vi "Test_Queue.vi"() -> (2 "Tests":cluster{"Test":string, "Passed":bool}[](array[cluster]), 3 "All Passed":bool)   [LabVIEW 2021]
uses:
  ebf6e7bd-4dea-41aa-a4d7-fcabb33fb88a.vi
  1f9cc325-9937-42ad-93f6-0991476be0d9.vi
  af2474c4-2a42-4373-a4e7-d7174c4c717d.vi
  fb02bb9d-60fe-4efe-999d-8fafea34c26a.vi
  86eb2c31-2ef4-4f52-8c7e-c4cd79eee94b.vi
  15bb192a-e047-4910-b6c7-e2d91b4fb920.vi
  e3e0b692-3f05-4cc3-bcdb-d52b2cb1c00c.vi
  07afb981-15fc-4acc-97a8-0c99b9836663.vi
  0269a72d-fd89-4c26-9187-e43185b182b9.vi
  803f4470-47be-4643-a591-48d54bf1cc4c.vi
  ec5fa7b9-9761-43ce-ad51-dc8d7309023d.vi
  7d11f8f4-9aa5-40e4-88f9-cf15113ac809.vi
  a4e05b25-b2fd-4a62-9474-6c8b1c6ba464.vi
  3a933310-1996-4eb1-bb35-2cef4bbc9920.vi
  3fbf7aaa-d5ae-4bec-ab0e-4ac27ad070b2.vi
  f4553291-fa86-418b-b39e-46cdf70e043e.vi
  b3874ef4-d7c0-4545-bae3-25086f4fe7ad.vi
  1ab1bd47-603c-456c-b9d0-96944e88f92c.vi
  ebbe48c1-b72b-4de3-aeb3-ba80bb7d0d19.vi
  8bdc6467-f6e5-4f75-9ac6-95094b1edd2b.vi
  35eb1fc5-534c-4ae0-b18f-a29eee8d1686.vi
  14dfade2-853f-44e8-b475-1791b1f25eec.vi
  4af17a5a-468f-4981-8f40-38f2c589f87d.vi
  fafea8c6-e71b-47bf-8fdc-74539dc463ec.vi
  be416df7-4f26-4020-a28b-5e551047e503.vi
  8d7d29ec-df87-4bcc-9fa1-3aa083bb282c.vi
  6a558a1d-279f-4cd8-a1d4-0ce029900aa4.vi
  7b643780-0266-49a5-bff5-7ddf02e75eca.vi
  b89bb2c3-d50e-4ca1-96dc-4f6891fa975b.vi
  f7c266ed-5b2f-4925-8a7e-d3378c7bde95.vi
  22155a5e-7ba0-482a-9fa4-40093b810291.vi
  <vilib>/Utility/error.llb/Error Cluster From Error Code.vi
  src/SubVIs/Map.vi
  src/Queue.lvlib
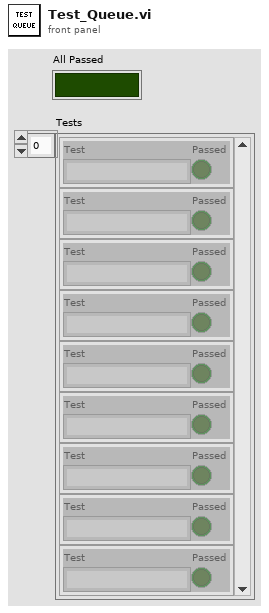
[diagram p1: front panel]
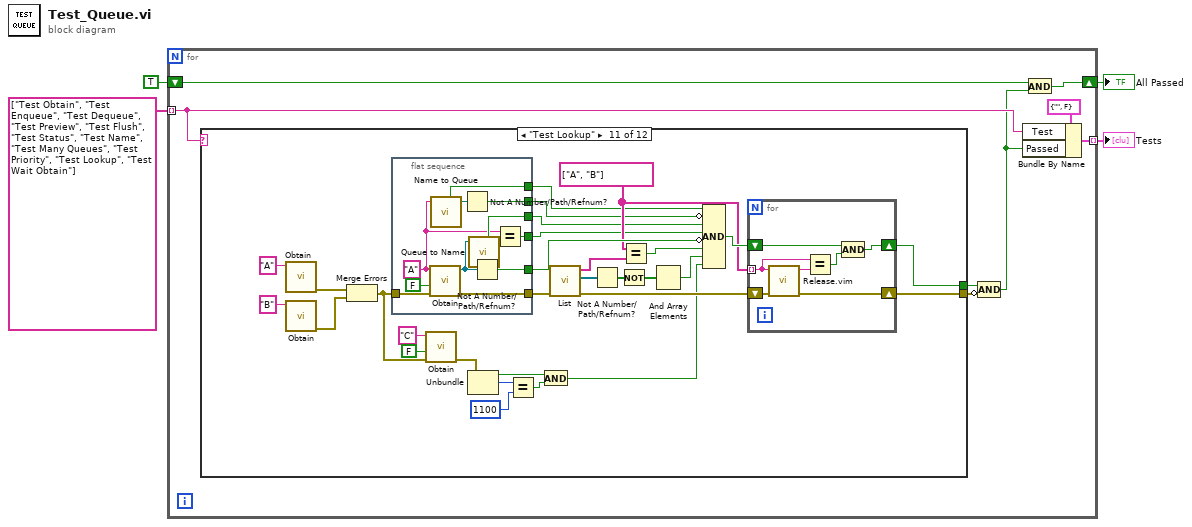
[diagram p0: block diagram]
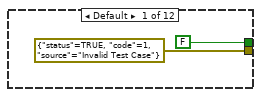
[diagram p2: hidden frame]
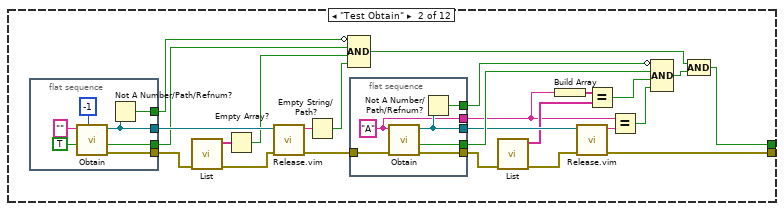
[diagram p3: hidden frame]
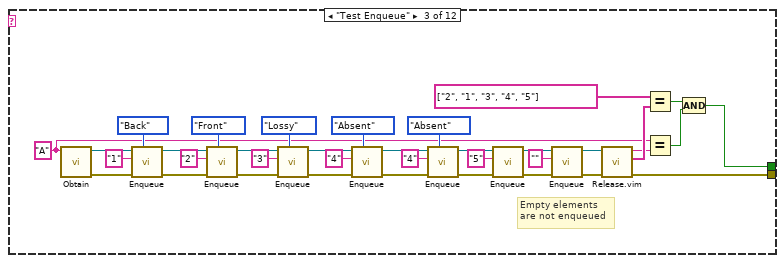
[diagram p4: hidden frame]
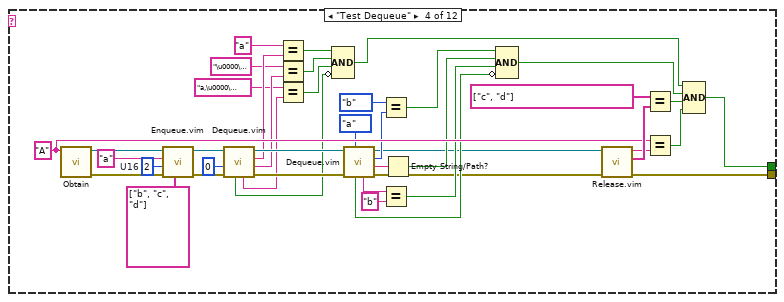
[diagram p5: hidden frame]
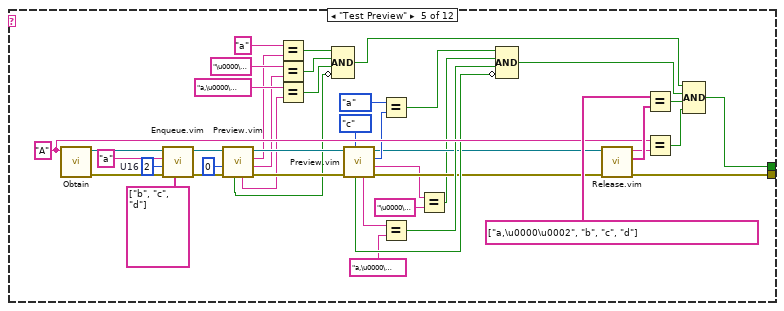
[diagram p6: hidden frame]
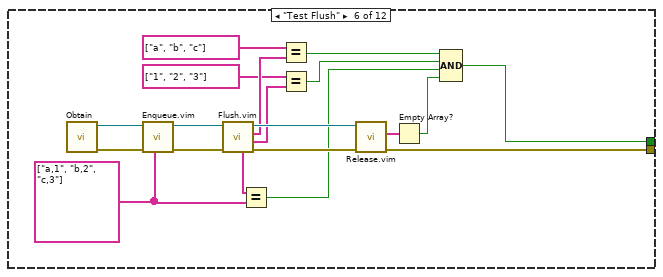
[diagram p7: hidden frame]
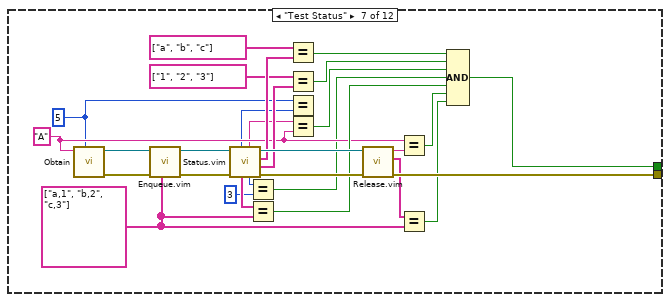
[diagram p8: hidden frame]
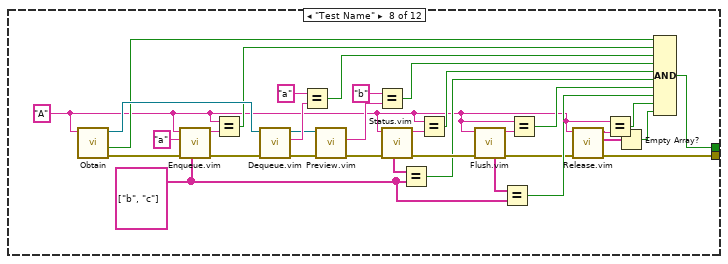
[diagram p9: hidden frame]
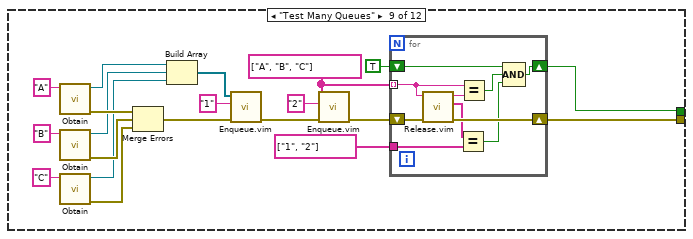
[diagram p10: hidden frame]
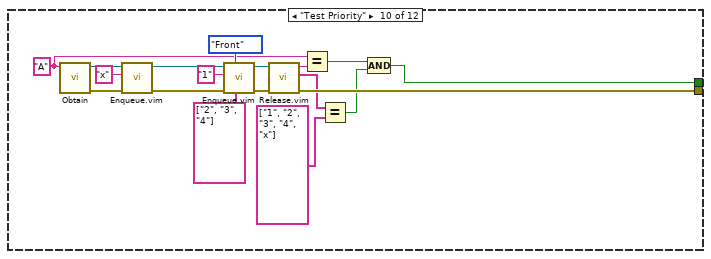
[diagram p11: hidden frame]
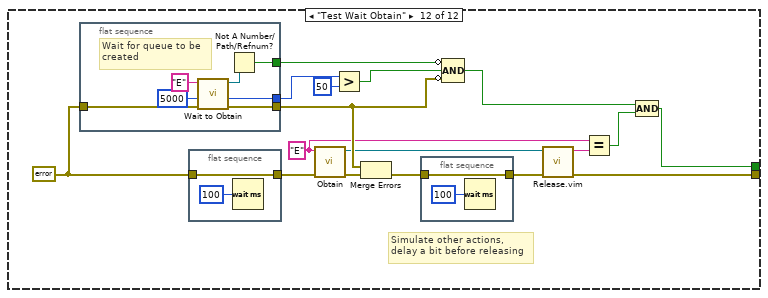
[diagram p12: hidden frame]
diagram:
  n1 = for {
    tunnel: string[] ["Test Obtain", "Test Enqueue", "Test Dequeue", "Test Preview", "Test Flush", "Test Status", "Test Name", "Test Many Queues", "Test Priority", "Test Lookup", "Test Wait Obtain"] -> [w8] mode=indexing
    shift-right: [w10] -> w2
    shift-left: TRUE -> [w11]
    tunnel: [w9] -> w1 mode=indexing
    n2 = case shown="\"Test Lookup\"" w8 {
      tunnel: [FALSE w30 w64 w126 w169 w180 w213 w222 w256 w291 w331 w358] -> w7
      tunnel: [errorcluster {"status"=TRUE, "code"=1, "source"="Invalid Test Case"} ("error in (no error)") w29 w67 w129 w172 w192 w221 w223 w260 w298 w333 w363] -> w5
      frame Default {
      }
      frame "Test Obtain" {
        n3 = flat-sequence {
          tunnel: [w52] -> w24
          tunnel: [w50] -> w39
          tunnel: [w49] -> w38
          tunnel: [w48] -> w37
          frame #0 {
            n4 = call "Obtain.vi"("Max Size (-1=Unlimited)"=-1, "Create if not Found? (T)"=TRUE, "Queue Name (\"\"=Unnamed)"="" ("Queue Name (\"\"=Unnamed)")) -> ("error out"=w52:errorcluster, "Created New?"=w48:bool, "Queue out"=w50:refnum<queue>)  [unwired: 6 in]
            n5 = Not A Number/Path/Refnum?(number/path/refnum=w50) -> (NaN/Path/Refnum?=w49:bool)
          }
        }
        n6 = call "List.vi"("error in (no error)"=w24) -> ("error out"=w23:errorcluster, "Queue Names"=w22:string[])  [unwired: 8 in, 1 out]
        n7 = Empty Array?(array=w22) -> (empty?=w21:bool)
        n8 = call "Release.vim"("error in (no error)"=w23, "Queue in"=w39) -> ("error out"=w33:errorcluster, "Queue Name"=w26:string)  [unwired: 7 in, 1 out]
        n9 = Empty String/Path?(string/path=w26) -> (empty?=w25:bool)
        n10 = Compound Arithmetic op=AND(invert w38, w37, w21, w25) -> (w31:bool)
        n11 = flat-sequence {
          tunnel: [w45] -> w36
          tunnel: [w44] -> w35
          tunnel: [w43] -> w34
          tunnel: [w42] -> w20
          tunnel: w33 -> [w41]
          tunnel: [w40] -> w16
          frame #0 {
            w40 = "A" ("Queue Name (\"\"=Unnamed)")
            n12 = call "Obtain.vi"("error in (no error)"=w41, "Queue Name (\"\"=Unnamed)"=w40) -> ("error out"=w42:errorcluster, "Created New?"=w45:bool, "Queue out"=w43:refnum<queue>)  [unwired: 7 in]
            n13 = Not A Number/Path/Refnum?(number/path/refnum=w43) -> (NaN/Path/Refnum?=w44:bool)
          }
        }
        n14 = call "List.vi"("error in (no error)"=w20) -> ("error out"=w19:errorcluster, "Queue Names"=w18:string[])  [unwired: 8 in, 1 out]
        n15 = Build Array(w16) -> (w17:string[])
        n16 = call "Release.vim"("error in (no error)"=w19, "Queue in"=w34) -> ("error out"=w29:errorcluster, "Queue Name"=w28:string)  [unwired: 7 in, 1 out]
        n17 = Equal?(x=w17, y=w18) -> (x = y?=w15:bool)
        n18 = Equal?(x=w16, y=w28) -> (x = y?=w27:bool)
        n19 = Compound Arithmetic op=AND(invert w35, w36, w15, w27) -> (w32:bool)
        n20 = Compound Arithmetic op=AND(w31, w32) -> (w30:bool)
      }
      frame "Test Enqueue" {
        w61 = "A" ("Queue Name (\"\"=Unnamed)")
        # "Empty elements\nare not enqueued"
        n21 = call "Obtain.vi"("Queue Name (\"\"=Unnamed)"=w61) -> ("error out"=w87:errorcluster, "Queue out"=w88:refnum<queue>)  [unwired: 8 in, 1 out]
        n22 = call "Enqueue.vi"("Method (Back)"=enum8{"Back", "Front", "Lossy", "Absent"}."Back", "error in (no error)"=w87, "Element"="1", "Queue in"=w88) -> ("error out"=w81:errorcluster, "Queue out"=w82:refnum<queue>)  [unwired: 6 in]
        n23 = call "Enqueue.vi"("Method (Back)"=enum8{"Back", "Front", "Lossy", "Absent"}."Front", "error in (no error)"=w81, "Element"="2", "Queue in"=w82) -> ("error out"=w77:errorcluster, "Queue out"=w78:refnum<queue>)  [unwired: 6 in]
        n24 = call "Enqueue.vi"("Method (Back)"=enum8{"Back", "Front", "Lossy", "Absent"}."Lossy", "error in (no error)"=w77, "Element"="3", "Queue in"=w78) -> ("error out"=w73:errorcluster, "Queue out"=w74:refnum<queue>)  [unwired: 6 in]
        n25 = call "Enqueue.vi"("Method (Back)"=enum8{"Back", "Front", "Lossy", "Absent"}."Absent", "error in (no error)"=w73, "Element"="4", "Queue in"=w74) -> ("error out"=w69:errorcluster, "Queue out"=w70:refnum<queue>)  [unwired: 6 in]
        n26 = call "Enqueue.vi"("Method (Back)"=enum8{"Back", "Front", "Lossy", "Absent"}."Absent", "error in (no error)"=w69, "Element"="4", "Queue in"=w70) -> ("error out"=w59:errorcluster, "Queue out"=w60:refnum<queue>)  [unwired: 6 in]
        n27 = call "Enqueue.vi"("error in (no error)"=w59, "Element"="5", "Queue in"=w60) -> ("error out"=w56:errorcluster, "Queue out"=w57:refnum<queue>)  [unwired: 7 in]
        n28 = call "Enqueue.vi"("error in (no error)"=w56, "Element"="", "Queue in"=w57) -> ("error out"=w55:errorcluster, "Queue out"=w54:refnum<queue>)  [unwired: 7 in]
        n29 = call "Release.vim"("error in (no error)"=w55, "Queue in"=w54) -> ("error out"=w67:errorcluster, "Remaining Elements"=w66:string[], "Queue Name"=w63:string)  [unwired: 7 in]
        n30 = Equal?(x=string[] ["2", "1", "3", "4", "5"] ("y"), y=w66) -> (x = y?=w65:bool)
        n31 = Equal?(x=w61, y=w63) -> (x = y?=w62:bool)
        n32 = Compound Arithmetic op=AND(w65, w62) -> (w64:bool)
      }
      frame "Test Dequeue" {
        w119 = u16 2  # U16
        w123 = "A" ("Queue Name (\"\"=Unnamed)")
        n33 = call "Obtain.vi"("Queue Name (\"\"=Unnamed)"=w123) -> ("error out"=w121:errorcluster, "Queue out"=w122:refnum<queue>)  [unwired: 8 in, 1 out]
        n34 = call "Enqueue.vim"("Messages"=string[] ["b", "c", "d"], "error in (no error)"=w121, "Data"=w119, "Message"="a", "Queue in"=w122) -> ("error out"=w117:errorcluster, "Queue out"=w116:refnum<queue>)  [unwired: 5 in]
        n35 = call "Dequeue.vim"("error in (no error)"=w117, "Timeout in ms (-1)"=0, "Queue in"=w116) -> ("error out"=w114:errorcluster, "Data"=w110:string, "Message"=w112:string, "Queue out"=w113:refnum<queue>, "Element"=w105:string, "Timed Out?"=w103:bool)  [unwired: 3 in]
        n36 = Equal?(x="a", y=w112) -> (x = y?=w108:bool)
        n37 = Equal?(x="\u0000\u0002", y=w110) -> (x = y?=w107:bool)
        n38 = Equal?(x="a,\u0000\u0002", y=w105) -> (x = y?=w104:bool)
        n39 = Compound Arithmetic op=AND(w108, w107, w104, invert w103) -> (w89:bool)
        n40 = call "Dequeue.vim"("Message Type"=enum16{"a", "b", "c", "d"}."a", "error in (no error)"=w114, "Queue in"=w113) -> ("error out"=w92:errorcluster, "Data"=w98:string, "Message"=w101:enum16{"a", "b", "c", "d"}, "Queue out"=w91:refnum<queue>, "Element"=w96:string, "Timed Out?"=w93:bool)  [unwired: 3 in]
        n41 = Equal?(x=enum16{"a", "b", "c", "d"}."b", y=w101) -> (x = y?=w99:bool)
        n42 = Equal?(x=w96, y="b") -> (x = y?=w94:bool)
        n43 = Empty String/Path?(string/path=w98) -> (empty?=w97:bool)
        n44 = Compound Arithmetic op=AND(w99, w97, w94, invert w93) -> (w90:bool)
        n45 = call "Release.vim"("error in (no error)"=w92, "Queue in"=w91) -> ("error out"=w129:errorcluster, "Remaining Elements"=w128:string[], "Queue Name"=w125:string)  [unwired: 7 in]
        n46 = Equal?(x=string[] ["c", "d"] ("y"), y=w128) -> (x = y?=w127:bool)
        n47 = Equal?(x=w123, y=w125) -> (x = y?=w124:bool)
        n48 = Compound Arithmetic op=AND(w89, w90, w127, w124) -> (w126:bool)
      }
      frame "Test Preview" {
        w162 = u16 2  # U16
        w166 = "A" ("Queue Name (\"\"=Unnamed)")
        n49 = call "Obtain.vi"("Queue Name (\"\"=Unnamed)"=w166) -> ("error out"=w164:errorcluster, "Queue out"=w165:refnum<queue>)  [unwired: 8 in, 1 out]
        n50 = call "Enqueue.vim"("Messages"=string[] ["b", "c", "d"], "error in (no error)"=w164, "Data"=w162, "Message"="a", "Queue in"=w165) -> ("error out"=w143:errorcluster, "Queue out"=w142:refnum<queue>)  [unwired: 5 in]
        n51 = call "Preview.vim"("error in (no error)"=w143, "Timeout in ms (-1)"=0, "Queue in"=w142) -> ("error out"=w140:errorcluster, "Data"=w136:string, "Message"=w135:string, "Queue out"=w141:refnum<queue>, "Element"=w138:string, "Timed Out?"=w137:bool)  [unwired: 3 in]
        n52 = Equal?(x="a", y=w135) -> (x = y?=w158:bool)
        n53 = Equal?(x="\u0000\u0002", y=w136) -> (x = y?=w157:bool)
        n54 = Equal?(x="a,\u0000\u0002", y=w138) -> (x = y?=w155:bool)
        n55 = Compound Arithmetic op=AND(w158, w157, w155, invert w137) -> (w144:bool)
        n56 = call "Preview.vim"("Message Type"=enum16{"a", "b", "c", "d"}."c", "error in (no error)"=w140, "Queue in"=w141) -> ("error out"=w147:errorcluster, "Data"=w132:string, "Message"=w153:enum16{"a", "b", "c", "d"}, "Queue out"=w146:refnum<queue>, "Element"=w150:string, "Timed Out?"=w148:bool)  [unwired: 3 in]
        n57 = Equal?(x=enum16{"a", "b", "c", "d"}."a", y=w153) -> (x = y?=w151:bool)
        n58 = Equal?(x=w150, y="a,\u0000\u0002" ("x")) -> (x = y?=w149:bool)
        n59 = Equal?(x=w132, y="\u0000\u0002" ("x")) -> (x = y?=w131:bool)
        n60 = Compound Arithmetic op=AND(w151, w131, w149, invert w148) -> (w145:bool)
        n61 = call "Release.vim"("error in (no error)"=w147, "Queue in"=w146) -> ("error out"=w172:errorcluster, "Remaining Elements"=w171:string[], "Queue Name"=w168:string)  [unwired: 7 in]
        n62 = Equal?(x=string[] ["a,\u0000\u0002", "b", "c", "d"] ("y"), y=w171) -> (x = y?=w170:bool)
        n63 = Equal?(x=w166, y=w168) -> (x = y?=w167:bool)
        n64 = Compound Arithmetic op=AND(w144, w145, w170, w167) -> (w169:bool)
      }
      frame "Test Flush" {
        w184 = string[] ["a,1", "b,2", "c,3"] ("Messages")
        n65 = call "Obtain.vi"() -> ("error out"=w188:errorcluster, "Queue out"=w189:refnum<queue>)  [unwired: 9 in, 1 out]
        n66 = call "Enqueue.vim"("Messages"=w184, "error in (no error)"=w188, "Queue in"=w189) -> ("error out"=w186:errorcluster, "Queue out"=w187:refnum<queue>)  [unwired: 7 in]
        n67 = call "Flush.vim"("error in (no error)"=w186, "Queue in"=w187) -> ("error out"=w191:errorcluster, "Data"=w176:string[], "Messages"=w179:string[], "Queue out"=w190:refnum<queue>, "Elements"=w185:string[])  [unwired: 5 in]
        n68 = Equal?(x=w185, y=w184) -> (x = y?=w181:bool)
        n69 = Equal?(x=string[] ["a", "b", "c"], y=w179) -> (x = y?=w174:bool)
        n70 = Equal?(x=string[] ["1", "2", "3"], y=w176) -> (x = y?=w175:bool)
        n71 = call "Release.vim"("error in (no error)"=w191, "Queue in"=w190) -> ("error out"=w192:errorcluster, "Remaining Elements"=w183:string[])  [unwired: 7 in, 1 out]
        n72 = Empty Array?(array=w183) -> (empty?=w182:bool)
        n73 = Compound Arithmetic op=AND(w174, w175, w181, w182) -> (w180:bool)
      }
      frame "Test Status" {
        w197 = 5 ("Max Size (-1=Unlimited)")
        w201 = "A" ("Queue Name (\"\"=Unnamed)")
        w204 = string[] ["a,1", "b,2", "c,3"] ("Messages")
        n74 = call "Obtain.vi"("Max Size (-1=Unlimited)"=w197, "Queue Name (\"\"=Unnamed)"=w201) -> ("error out"=w217:errorcluster, "Queue out"=w218:refnum<queue>)  [unwired: 7 in, 1 out]
        n75 = call "Enqueue.vim"("Messages"=w204, "error in (no error)"=w217, "Queue in"=w218) -> ("error out"=w215:errorcluster, "Queue out"=w216:refnum<queue>)  [unwired: 7 in]
        n76 = call "Status.vim"("error in (no error)"=w215, "Queue in"=w216) -> ("error out"=w220:errorcluster, "Data"=w209:string[], "Messages"=w212:string[], "Queue out"=w219:refnum<queue>, "# Elements in Queue"=w196:i32, "Queue Name"=w200:string, "Elements"=w206:string[], "Max Size"=w198:i32)  [unwired: 2 in]
        n77 = Equal?(x=w196, y=3) -> (x = y?=w194:bool)
        n78 = Equal?(x=w206, y=w204) -> (x = y?=w214:bool)
        n79 = Equal?(x=string[] ["a", "b", "c"], y=w212) -> (x = y?=w207:bool)
        n80 = Equal?(x=string[] ["1", "2", "3"], y=w209) -> (x = y?=w208:bool)
        n81 = Equal?(x=w197, y=w198) -> ()  [unwired: 1 out]
        n82 = Equal?(x=w200, y=w201) -> (x = y?=w199:bool)
        n83 = call "Release.vim"("error in (no error)"=w220, "Queue in"=w219) -> ("error out"=w221:errorcluster, "Remaining Elements"=w205:string[], "Queue Name"=w202:string)  [unwired: 7 in]
        n84 = Equal?(x=w201, y=w202) -> (x = y?=w193:bool)
        n85 = Equal?(x=w205, y=w204) -> (x = y?=w203:bool)
        n86 = Compound Arithmetic op=AND(w207, w208, w199, w194, w214, w193, w203) -> (w213:bool)
      }
      frame "Test Name" {
        w232 = string[] ["b", "c"] ("Messages")
        w227 = "A" ("Queue Name (\"\"=Unnamed)")
        n87 = call "Obtain.vi"("Queue Name (\"\"=Unnamed)"=w227) -> ("error out"=w255:errorcluster, "Created New?"=w248:bool, "Queue out"=w252:refnum<queue>)  [unwired: 8 in]
        n88 = call "Enqueue.vim"("Messages"=w232, "error in (no error)"=w255, "Message"="a", "Queue in"=w227) -> ("error out"=w253:errorcluster, "Queue out"=w238:string)  [unwired: 6 in]
        n89 = Equal?(x=w227, y=w238) -> (x = y?=w237:bool)
        n90 = call "Dequeue.vim"("error in (no error)"=w253, "Queue in"=w252) -> ("error out"=w247:errorcluster, "Message"=w251:string, "Queue out"=w246:refnum<queue>)  [unwired: 4 in, 3 out]
        n91 = Equal?(x="a", y=w251) -> (x = y?=w249:bool)
        n92 = call "Preview.vim"("error in (no error)"=w247, "Queue in"=w246) -> ("error out"=w242:errorcluster, "Message"=w244:string)  [unwired: 4 in, 4 out]
        n93 = Equal?(x="b", y=w244) -> (x = y?=w243:bool)
        n94 = call "Status.vim"("error in (no error)"=w242, "Queue in"=w227) -> ("error out"=w241:errorcluster, "Queue out"=w240:string, "Elements"=w236:string[])  [unwired: 2 in, 5 out]
        n95 = Equal?(x=w236, y=w232) -> (x = y?=w234:bool)
        n96 = Equal?(x=w227, y=w240) -> (x = y?=w235:bool)
        n97 = call "Flush.vim"("error in (no error)"=w241, "Queue in"=w227) -> ("error out"=w229:errorcluster, "Queue out"=w239:string, "Elements"=w233:string[])  [unwired: 5 in, 2 out]
        n98 = Equal?(x=w233, y=w232) -> (x = y?=w230:bool)
        n99 = Equal?(x=w227, y=w239) -> (x = y?=w231:bool)
        n100 = call "Release.vim"("error in (no error)"=w229, "Queue in"=w227) -> ("error out"=w223:errorcluster, "Remaining Elements"=w225:string[], "Queue Name"=w228:string)  [unwired: 7 in]
        n101 = Equal?(x=w227, y=w228) -> (x = y?=w226:bool)
        n102 = Empty Array?(array=w225) -> (empty?=w224:bool)
        n103 = Compound Arithmetic op=AND(w248, w237, w249, w243, w235, w234, w231, w230, w226, w224) -> (w222:bool)
      }
      frame "Test Many Queues" {
        w259 = string[] ["A", "B", "C"]
        n104 = call "Obtain.vi"("Queue Name (\"\"=Unnamed)"="A" ("Queue Name (\"\"=Unnamed)")) -> ("error out"=w272:errorcluster, "Queue out"=w265:refnum<queue>)  [unwired: 8 in, 1 out]
        n105 = call "Obtain.vi"("Queue Name (\"\"=Unnamed)"="B" ("Queue Name (\"\"=Unnamed)")) -> ("error out"=w273:errorcluster, "Queue out"=w264:refnum<queue>)  [unwired: 8 in, 1 out]
        n106 = call "Obtain.vi"("Queue Name (\"\"=Unnamed)"="C" ("Queue Name (\"\"=Unnamed)")) -> ("error out"=w270:errorcluster, "Queue out"=w263:refnum<queue>)  [unwired: 8 in, 1 out]
        n107 = Merge Errors(w272, w273, w270) -> (w267:errorcluster)
        n108 = Build Array(w265, w264, w263) -> (w262:refnum<queue>[])
        n109 = call "Enqueue.vim"("error in (no error)"=w267, "Message"="1", "Queue in"=w262) -> ("error out"=w266:errorcluster)  [unwired: 7 in, 1 out]
        n110 = call "Enqueue.vim"("error in (no error)"=w266, "Message"="2", "Queue in"=w259) -> ("error out"=w261:errorcluster)  [unwired: 7 in, 1 out]
        n111 = for {
          shift-right: [w284] -> w260
          shift-left: w261 -> [w285]
          tunnel: w259 -> [w282] mode=indexing
          tunnel: string[] ["1", "2"] ("y") -> [w280]
          shift-right: [w277] -> w256
          shift-left: TRUE -> [w276]
          n112 = call "Release.vim"("error in (no error)"=w285, "Queue in"=w282) -> ("error out"=w284:errorcluster, "Remaining Elements"=w281:string[], "Queue Name"=w283:string)  [unwired: 7 in]
          n113 = Equal?(x=w281, y=w280) -> (x = y?=w278:bool)
          n114 = Equal?(x=w282, y=w283) -> (x = y?=w279:bool)
          n115 = Compound Arithmetic op=AND(w276, w279, w278) -> (w277:bool)
        }
      }
      frame "Test Priority" {
        w295 = "A" ("Queue Name (\"\"=Unnamed)")
        n116 = call "Obtain.vi"("Queue Name (\"\"=Unnamed)"=w295) -> ("error out"=w289:errorcluster, "Queue out"=w290:refnum<queue>)  [unwired: 8 in, 1 out]
        n117 = call "Enqueue.vim"("error in (no error)"=w289, "Message"="x", "Queue in"=w290) -> ("error out"=w288:errorcluster, "Queue out"=w287:refnum<queue>)  [unwired: 7 in]
        n118 = call "Enqueue.vim"("Messages"=string[] ["2", "3", "4"], "Method (Back)"=enum8{"Back", "Front", "Lossy", "Absent"}."Front", "error in (no error)"=w288, "Message"="1", "Queue in"=w287) -> ("error out"=w300:errorcluster, "Queue out"=w299:refnum<queue>)  [unwired: 5 in]
        n119 = call "Release.vim"("error in (no error)"=w300, "Queue in"=w299) -> ("error out"=w298:errorcluster, "Remaining Elements"=w297:string[], "Queue Name"=w296:string)  [unwired: 7 in]
        n120 = Equal?(x=w295, y=w296) -> (x = y?=w293:bool)
        n121 = Equal?(x=w297, y=string[] ["1", "2", "3", "4", "x"]) -> (x = y?=w292:bool)
        n122 = Compound Arithmetic op=AND(w293, w292) -> (w291:bool)
      }
      frame "Test Lookup" {
        w308 = string[] ["A", "B"] ("y")
        n123 = call "Obtain.vi"("Queue Name (\"\"=Unnamed)"="A" ("Queue Name (\"\"=Unnamed)")) -> ("error out"=w330:errorcluster)  [unwired: 8 in, 2 out]
        n124 = call "Obtain.vi"("Queue Name (\"\"=Unnamed)"="B" ("Queue Name (\"\"=Unnamed)")) -> ("error out"=w328:errorcluster)  [unwired: 8 in, 2 out]
        n125 = Merge Errors(w330, w328) -> (w325:errorcluster)
        n126 = flat-sequence {
          tunnel: w325 -> [w351]
          tunnel: [w350] -> w319
          tunnel: [w349] -> w318
          tunnel: [w347] -> w307
          tunnel: [w346] -> w306
          tunnel: [w344] -> w305
          tunnel: [w341] -> w304
          frame #0 {
            w342 = "A" ("Queue Name (\"\"=Unnamed)")
            n127 = call "Obtain.vi"("error in (no error)"=w351, "Create if not Found? (T)"=FALSE, "Queue Name (\"\"=Unnamed)"=w342) -> ("error out"=w349:errorcluster, "Queue out"=w345:refnum<queue>)  [unwired: 6 in, 1 out]
            n128 = call "Name to Queue.vi"("Queue Name in"=w342) -> ("Found?"=w346:bool, "Queue out"=w348:refnum<queue>)  [unwired: 7 in]
            n129 = Not A Number/Path/Refnum?(number/path/refnum=w348) -> (NaN/Path/Refnum?=w347:bool)
            n130 = call "Queue to Name.vi"("Queue in"=w345) -> ("Found?"=w344:bool, "Queue Name out"=w343:string)  [unwired: 7 in]
            n131 = Not A Number/Path/Refnum?(number/path/refnum=w345) -> (NaN/Path/Refnum?=w350:bool)
            n132 = Equal?(x=w342, y=w343) -> (x = y?=w341:bool)
          }
        }
        n133 = call "Obtain.vi"("error in (no error)"=w325, "Create if not Found? (T)"=FALSE, "Queue Name (\"\"=Unnamed)"="C" ("Queue Name (\"\"=Unnamed)")) -> ("error out"=w324:errorcluster)  [unwired: 6 in, 2 out]
        n134 = Unbundle(w324) -> ("status"=w322:bool, "code"=w323:i32)  [unwired: 1 out]
        n135 = Equal?(x=w323, y=1100) -> (x = y?=w321:bool)
        n136 = And(x=w322, y=w321) -> (x .and. y?=w315:bool)
        n137 = call "List.vi"("error in (no error)"=w318) -> ("error out"=w316:errorcluster, "Queues"=w313:refnum<queue>[], "Queue Names"=w314:string[])  [unwired: 8 in]
        n138 = Not A Number/Path/Refnum?(number/path/refnum=w313) -> (NaN/Path/Refnum?=w312:bool[])
        n139 = Not(x=w312) -> (.not. x?=w311:bool[])
        n140 = Equal?(x=w308, y=w314) -> (x = y?=w317:bool)
        n141 = And Array Elements(Boolean array=w311) -> (logical AND=w310:bool)
        n142 = Compound Arithmetic op=AND(w306, invert w307, w305, w304, invert w319, w317, w310, w315) -> (w309:bool)
        n143 = for {
          shift-right: [w340] -> w333
          shift-left: w316 -> [w336]
          shift-right: [w337] -> w331
          shift-left: w309 -> [w335]
          tunnel: w308 -> [w334] mode=indexing
          n144 = call "Release.vim"("error in (no error)"=w336, "Queue in"=w334) -> ("error out"=w340:errorcluster, "Queue Name"=w339:string)  [unwired: 7 in, 1 out]
          n145 = Equal?(x=w334, y=w339) -> (x = y?=w338:bool)
          n146 = Compound Arithmetic op=AND(w335, w338) -> (w337:bool)
        }
      }
      frame "Test Wait Obtain" {
        w369 = errorcluster {"status"=FALSE, "code"=0, "source"=""} ("error in (no error)")
        w361 = "E" ("Queue Name (\"\"=Unnamed)")
        # "Simulate other actions,\ndelay a bit before releasing"
        n147 = flat-sequence {
          tunnel: w369 -> [w377]
          tunnel: [w374] -> w367
          tunnel: [w373] -> w365
          tunnel: [w372] -> w357
          frame #0 {
            # "Wait for queue to be\ncreated"
            n148 = call "Wait to Obtain.vi"("error in (no error)"=w377, "Timeout in ms (5000)"=u32 5000, "Queue Name"="E") -> ("error out"=w373:errorcluster, "ms Elapsed"=w372:u32, "Queue out"=w375:refnum<queue>)  [unwired: 6 in]
            n149 = Not A Number/Path/Refnum?(number/path/refnum=w375) -> (NaN/Path/Refnum?=w374:bool)
          }
        }
        n150 = flat-sequence {
          tunnel: w369 -> [w379]
          tunnel: [w379] -> w368
          frame #0 {
            n151 = Wait (ms)(milliseconds to wait=u32 100) -> ()  [unwired: 1 out]
          }
        }
        n152 = call "Obtain.vi"("error in (no error)"=w368, "Queue Name (\"\"=Unnamed)"=w361) -> ("error out"=w366:errorcluster, "Queue out"=w364:refnum<queue>)  [unwired: 7 in, 1 out]
        n153 = Greater?(x=w357, y=u32 50) -> (0:w355:bool)
        n154 = Merge Errors(w365, w366) -> (w354:errorcluster)
        n155 = flat-sequence {
          tunnel: w354 -> [w370]
          tunnel: [w370] -> w353
          frame #0 {
            n156 = Wait (ms)(milliseconds to wait=u32 100) -> ()  [unwired: 1 out]
          }
        }
        n157 = Compound Arithmetic op=AND(invert w367, w355, invert w365) -> (w359:bool)
        n158 = call "Release.vim"("error in (no error)"=w353, "Queue in"=w364) -> ("error out"=w363:errorcluster, "Queue Name"=w362:string)  [unwired: 7 in, 1 out]
        n159 = Equal?(x=w361, y=w362) -> (x = y?=w360:bool)
        n160 = Compound Arithmetic op=AND(w359, w360) -> (w358:bool)
      }
    }
    n161 = Compound Arithmetic op=AND(w7, invert w5) -> (w6:bool)
    n162 = Bundle By Name(cluster=cluster{"Test":string, "Passed":bool} {"Test"="", "Passed"=FALSE} ("Cluster"), "Test"=w8, "Passed"=w6) -> (w9:cluster{"Test":string, "Passed":bool})
    n163 = And(x=w11, y=w6) -> (x .and. y?=w10:bool)
  }
  "All Passed" <- w2
  "Tests" <- w1
